vi "beta-3.1.0.vi"(5 "Load":bool, 6 "Configure":bool, 7 "Output Configuration":T2={"Channel0"={"function"=enum."OFF", "scan end"=3.5, "scan begin"=0.0, "scan step"=0.0, "main input"=enum."DIO0", "sub input"=enum."DIO0", "boolean low"=3.5, "boolean high"=0.0}, "Channel1"={"function"=enum."OFF", "scan end"=3.5, "scan begin"=0.0, "scan step"=0.0, "main input"=enum."DIO0", "sub input"=enum."DIO0", "boolean low"=3.5, "boolean high"=0.0}, "Channel2"={"function"=enum."OFF", "scan end"=3.5, "scan begin"=0.0, "scan step"=0.0, "main input"=enum."DIO0", "sub input"=enum."DIO0", "boolean low"=3.5, "boolean high"=0.0}, "Channel3"={"function"=enum."OFF", "scan end"=3.5, "scan begin"=0.0, "scan step"=0.0, "main input"=enum."DIO0", "sub input"=enum."DIO0", "boolean low"=3.5, "boolean high"=0.0}, "Channel4"={"function"=enum."OFF", "scan end"=3.5, "scan begin"=0.0, "scan step"=0.0, "main input"=enum."DIO0", "sub input"=enum."DIO0", "boolean low"=3.5, "boolean high"=0.0}, "Channel5"={"function"=enum."OFF", "scan end"=3.5, "scan begin"=0.0, "scan step"=0.0, "main input"=enum."DIO0", "sub input"=enum."DIO0", "boolean low"=3.5, "boolean high"=0.0}, "Channel6"={"function"=enum."OFF", "scan end"=3.5, "scan begin"=0.0, "scan step"=0.0, "main input"=enum."DIO0", "sub input"=enum."DIO0", "boolean low"=3.5, "boolean high"=0.0}, "Channel7"={"function"=enum."OFF", "scan end"=3.5, "scan begin"=0.0, "scan step"=0.0, "main input"=enum."DIO0", "sub input"=enum."DIO0", "boolean low"=3.5, "boolean high"=0.0}, "Channel8"={"function"=enum."OFF", "scan end"=3.5, "scan begin"=0.0, "scan step"=0.0, "main input"=enum."DIO0", "sub input"=enum."DIO0", "boolean low"=3.5, "boolean high"=0.0}, "Channel9"={"function"=enum."OFF", "scan end"=3.5, "scan begin"=0.0, "scan step"=0.0, "main input"=enum."DIO0", "sub input"=enum."DIO0", "boolean low"=3.5, "boolean high"=0.0}, "Channel10"={"function"=enum."OFF", "scan end"=3.5, "scan begin"=0.0, "scan step"=0.0, "main input"=enum."DIO0", "sub input"=enum."DIO0", "boolean low"=3.5, "boolean high"=0.0}, "Channel11"={"function"=enum."OFF", "scan end"=3.5, "scan begin"=0.0, "scan step"=0.0, "main input"=enum."DIO0", "sub input"=enum."DIO0", "boolean low"=3.5, "boolean high"=0.0}, "Channel12"={"function"=enum."OFF", "scan end"=3.5, "scan begin"=0.0, "scan step"=0.0, "main input"=enum."DIO0", "sub input"=enum."DIO0", "boolean low"=3.5, "boolean high"=0.0}, "Channel13"={"function"=enum."OFF", "scan end"=3.5, "scan begin"=0.0, "scan step"=0.0, "main input"=enum."DIO0", "sub input"=enum."DIO0", "boolean low"=3.5, "boolean high"=0.0}, "Channel14"={"function"=enum."OFF", "scan end"=3.5, "scan begin"=0.0, "scan step"=0.0, "main input"=enum."DIO0", "sub input"=enum."DIO0", "boolean low"=3.5, "boolean high"=0.0}, "Channel15"={"function"=enum."OFF", "scan end"=3.5, "scan begin"=0.0, "scan step"=0.0, "main input"=enum."DIO0", "sub input"=enum."DIO0", "boolean low"=3.5, "boolean high"=0.0}} {"Channel15"."boolean high" format="%#_17g"; "Channel15"."boolean low" format="%#_17g"; "Channel15"."scan step" format="%#_17g"; "Channel15"."scan begin" format="%#_17g"; "Channel15"."scan end" format="%#_17g"; "Channel14"."boolean high" format="%#_17g"; "Channel14"."boolean low" format="%#_17g"; "Channel14"."scan step" format="%#_17g"; "Channel14"."scan begin" format="%#_17g"; "Channel14"."scan end" format="%#_17g"; "Channel13"."boolean high" format="%#_17g"; "Channel13"."boolean low" format="%#_17g"; "Channel13"."scan step" format="%#_17g"; "Channel13"."scan begin" format="%#_17g"; "Channel13"."scan end" format="%#_17g"; "Channel12"."boolean high" format="%#_17g"; "Channel12"."boolean low" format="%#_17g"; "Channel12"."scan step" format="%#_17g"; "Channel12"."scan begin" format="%#_17g"; "Channel12"."scan end" format="%#_17g"; "Channel11"."boolean high" format="%#_17g"; "Channel11"."boolean low" format="%#_17g"; "Channel11"."scan step" format="%#_17g"; "Channel11"."scan begin" format="%#_17g"; "Channel11"."scan end" format="%#_17g"; "Channel10"."boolean high" format="%#_17g"; "Channel10"."boolean low" format="%#_17g"; "Channel10"."scan step" format="%#_17g"; "Channel10"."scan begin" format="%#_17g"; "Channel10"."scan end" format="%#_17g"; "Channel9"."boolean high" format="%#_17g"; "Channel9"."boolean low" format="%#_17g"; "Channel9"."scan step" format="%#_17g"; "Channel9"."scan begin" format="%#_17g"; "Channel9"."scan end" format="%#_17g"; "Channel8"."boolean high" format="%#_17g"; "Channel8"."boolean low" format="%#_17g"; "Channel8"."scan step" format="%#_17g"; "Channel8"."scan begin" format="%#_17g"; "Channel8"."scan end" format="%#_17g"; "Channel7"."boolean high" format="%#_17g"; "Channel7"."boolean low" format="%#_17g"; "Channel7"."scan step" format="%#_17g"; "Channel7"."scan begin" format="%#_17g"; "Channel7"."scan end" format="%#_17g"; "Channel6"."boolean high" format="%#_17g"; "Channel6"."boolean low" format="%#_17g"; "Channel6"."scan step" format="%#_17g"; "Channel6"."scan begin" format="%#_17g"; "Channel6"."scan end" format="%#_17g"; "Channel5"."boolean high" format="%#_17g"; "Channel5"."boolean low" format="%#_17g"; "Channel5"."scan step" format="%#_17g"; "Channel5"."scan begin" format="%#_17g"; "Channel5"."scan end" format="%#_17g"; "Channel4"."boolean high" format="%#_17g"; "Channel4"."boolean low" format="%#_17g"; "Channel4"."scan step" format="%#_17g"; "Channel4"."scan begin" format="%#_17g"; "Channel4"."scan end" format="%#_17g"; "Channel3"."boolean high" format="%#_17g"; "Channel3"."boolean low" format="%#_17g"; "Channel3"."scan step" format="%#_17g"; "Channel3"."scan begin" format="%#_17g"; "Channel3"."scan end" format="%#_17g"; "Channel2"."boolean high" format="%#_17g"; "Channel2"."boolean low" format="%#_17g"; "Channel2"."scan step" format="%#_17g"; "Channel2"."scan begin" format="%#_17g"; "Channel2"."scan end" format="%#_17g"; "Channel1"."boolean high" format="%#_17g"; "Channel1"."boolean low" format="%#_17g"; "Channel1"."scan step" format="%#_17g"; "Channel1"."scan begin" format="%#_17g"; "Channel1"."scan end" format="%#_17g"; "Channel0"."boolean high" format="%#_17g"; "Channel0"."boolean low" format="%#_17g"; "Channel0"."scan step" format="%#_17g"; "Channel0"."scan begin" format="%#_17g"; "Channel0"."scan end" format="%#_17g"}) -> (0 "State":enum16{"Loading", "Running"}(ring), 4 "change indicator":T1)   [LabVIEW 2016]
uses:
  <vilib>/FPGAPlugInAG/cRIO-9063/niLvFpga_Open_cRIO-9063.vi
  <vilib>/rvi/interface/common/dynamic/niFpgaDynamicAddResources.vi
  <vilib>/Utility/error.llb/Error Cluster From Error Code.vi
  <vilib>/rvi/errors/niLvFpgaAdjustHostInterfaceError.vi
  <vilib>/FPGAPlugInAG/Dynamic/niLvFpga_Close_Dynamic.vi
  <vilib>/rvi/interface/nirviOpenFPGA/nirviOpenFPGA.xnode
  FPGA Bitfiles/multi-functionpr_FPGATarget_multi-function-f_bsn-gyeHrfY.lvbitx
  <vilib>/rvi/interface/nirviReadWriteControl/nirviReadWriteControl.xnode
  <vilib>/rvi/interface/nirviCloseFPGA/nirviCloseFPGA.xnode
  NiFpgaLv.dll
  <vilib>/rvi/interface/Simulation/niFpgaSimulationCallBeginRW.vi
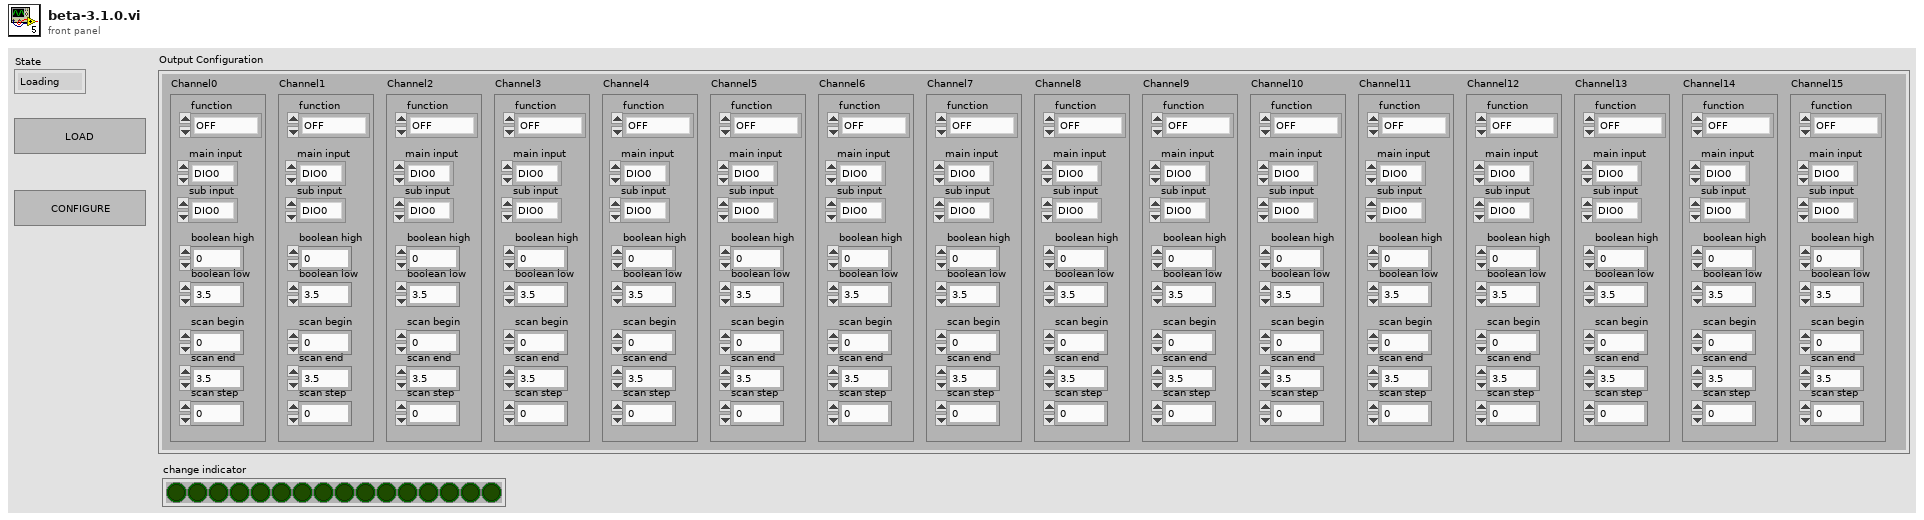
[diagram p1: front panel]
types:
  T1 = cluster{bool, bool, bool, bool, bool, bool, bool, bool, bool, bool, bool, bool, bool, bool, bool, bool}
  T2 = cluster{"Channel0":cluster{"function":enum16{"OFF", "SWITCH", "AND GATE", "OR GATE", "ITERATION"}, "scan end":sgl, "scan begin":sgl, "scan step":sgl, "main input":enum16{"DIO0", "DIO1", "DIO2", "DIO3", "DIO4", "DIO5", "DIO6", "DIO7", "DIO8", "DIO9", "DIO10", "DIO11", "DIO12", "DIO13", "DIO14", "DIO15", "DIO16", "DIO17", "DIO18", "DIO19", "DIO20", "DIO21", "DIO22", "DIO23", "DIO24", "DIO25", "DIO26", "DIO27", "DIO28", "DIO29", "DIO30", "DIO31"}, "sub input":enum16{"DIO0", "DIO1", "DIO2", "DIO3", "DIO4", "DIO5", "DIO6", "DIO7", "DIO8", "DIO9", "DIO10", "DIO11", "DIO12", "DIO13", "DIO14", "DIO15", "DIO16", "DIO17", "DIO18", "DIO19", "DIO20", "DIO21", "DIO22", "DIO23", "DIO24", "DIO25", "DIO26", "DIO27", "DIO28", "DIO29", "DIO30", "DIO31"}, "boolean low":sgl, "boolean high":sgl}, "Channel1":cluster{"function":enum16{"OFF", "SWITCH", "AND GATE", "OR GATE", "ITERATION"}, "scan end":sgl, "scan begin":sgl, "scan step":sgl, "main input":enum16{"DIO0", "DIO1", "DIO2", "DIO3", "DIO4", "DIO5", "DIO6", "DIO7", "DIO8", "DIO9", "DIO10", "DIO11", "DIO12", "DIO13", "DIO14", "DIO15", "DIO16", "DIO17", "DIO18", "DIO19", "DIO20", "DIO21", "DIO22", "DIO23", "DIO24", "DIO25", "DIO26", "DIO27", "DIO28", "DIO29", "DIO30", "DIO31"}, "sub input":enum16{"DIO0", "DIO1", "DIO2", "DIO3", "DIO4", "DIO5", "DIO6", "DIO7", "DIO8", "DIO9", "DIO10", "DIO11", "DIO12", "DIO13", "DIO14", "DIO15", "DIO16", "DIO17", "DIO18", "DIO19", "DIO20", "DIO21", "DIO22", "DIO23", "DIO24", "DIO25", "DIO26", "DIO27", "DIO28", "DIO29", "DIO30", "DIO31"}, "boolean low":sgl, "boolean high":sgl}, "Channel2":cluster{"function":enum16{"OFF", "SWITCH", "AND GATE", "OR GATE", "ITERATION"}, "scan end":sgl, "scan begin":sgl, "scan step":sgl, "main input":enum16{"DIO0", "DIO1", "DIO2", "DIO3", "DIO4", "DIO5", "DIO6", "DIO7", "DIO8", "DIO9", "DIO10", "DIO11", "DIO12", "DIO13", "DIO14", "DIO15", "DIO16", "DIO17", "DIO18", "DIO19", "DIO20", "DIO21", "DIO22", "DIO23", "DIO24", "DIO25", "DIO26", "DIO27", "DIO28", "DIO29", "DIO30", "DIO31"}, "sub input":enum16{"DIO0", "DIO1", "DIO2", "DIO3", "DIO4", "DIO5", "DIO6", "DIO7", "DIO8", "DIO9", "DIO10", "DIO11", "DIO12", "DIO13", "DIO14", "DIO15", "DIO16", "DIO17", "DIO18", "DIO19", "DIO20", "DIO21", "DIO22", "DIO23", "DIO24", "DIO25", "DIO26", "DIO27", "DIO28", "DIO29", "DIO30", "DIO31"}, "boolean low":sgl, "boolean high":sgl}, "Channel3":cluster{"function":enum16{"OFF", "SWITCH", "AND GATE", "OR GATE", "ITERATION"}, "scan end":sgl, "scan begin":sgl, "scan step":sgl, "main input":enum16{"DIO0", "DIO1", "DIO2", "DIO3", "DIO4", "DIO5", "DIO6", "DIO7", "DIO8", "DIO9", "DIO10", "DIO11", "DIO12", "DIO13", "DIO14", "DIO15", "DIO16", "DIO17", "DIO18", "DIO19", "DIO20", "DIO21", "DIO22", "DIO23", "DIO24", "DIO25", "DIO26", "DIO27", "DIO28", "DIO29", "DIO30", "DIO31"}, "sub input":enum16{"DIO0", "DIO1", "DIO2", "DIO3", "DIO4", "DIO5", "DIO6", "DIO7", "DIO8", "DIO9", "DIO10", "DIO11", "DIO12", "DIO13", "DIO14", "DIO15", "DIO16", "DIO17", "DIO18", "DIO19", "DIO20", "DIO21", "DIO22", "DIO23", "DIO24", "DIO25", "DIO26", "DIO27", "DIO28", "DIO29", "DIO30", "DIO31"}, "boolean low":sgl, "boolean high":sgl}, "Channel4":cluster{"function":enum16{"OFF", "SWITCH", "AND GATE", "OR GATE", "ITERATION"}, "scan end":sgl, "scan begin":sgl, "scan step":sgl, "main input":enum16{"DIO0", "DIO1", "DIO2", "DIO3", "DIO4", "DIO5", "DIO6", "DIO7", "DIO8", "DIO9", "DIO10", "DIO11", "DIO12", "DIO13", "DIO14", "DIO15", "DIO16", "DIO17", "DIO18", "DIO19", "DIO20", "DIO21", "DIO22", "DIO23", "DIO24", "DIO25", "DIO26", "DIO27", "DIO28", "DIO29", "DIO30", "DIO31"}, "sub input":enum16{"DIO0", "DIO1", "DIO2", "DIO3", "DIO4", "DIO5", "DIO6", "DIO7", "DIO8", "DIO9", "DIO10", "DIO11", "DIO12", "DIO13", "DIO14", "DIO15", "DIO16", "DIO17", "DIO18", "DIO19", "DIO20", "DIO21", "DIO22", "DIO23", "DIO24", "DIO25", "DIO26", "DIO27", "DIO28", "DIO29", "DIO30", "DIO31"}, "boolean low":sgl, "boolean high":sgl}, "Channel5":cluster{"function":enum16{"OFF", "SWITCH", "AND GATE", "OR GATE", "ITERATION"}, "scan end":sgl, "scan begin":sgl, "scan step":sgl, "main input":enum16{"DIO0", "DIO1", "DIO2", "DIO3", "DIO4", "DIO5", "DIO6", "DIO7", "DIO8", "DIO9", "DIO10", "DIO11", "DIO12", "DIO13", "DIO14", "DIO15", "DIO16", "DIO17", "DIO18", "DIO19", "DIO20", "DIO21", "DIO22", "DIO23", "DIO24", "DIO25", "DIO26", "DIO27", "DIO28", "DIO29", "DIO30", "DIO31"}, "sub input":enum16{"DIO0", "DIO1", "DIO2", "DIO3", "DIO4", "DIO5", "DIO6", "DIO7", "DIO8", "DIO9", "DIO10", "DIO11", "DIO12", "DIO13", "DIO14", "DIO15", "DIO16", "DIO17", "DIO18", "DIO19", "DIO20", "DIO21", "DIO22", "DIO23", "DIO24", "DIO25", "DIO26", "DIO27", "DIO28", "DIO29", "DIO30", "DIO31"}, "boolean low":sgl, "boolean high":sgl}, "Channel6":cluster{"function":enum16{"OFF", "SWITCH", "AND GATE", "OR GATE", "ITERATION"}, "scan end":sgl, "scan begin":sgl, "scan step":sgl, "main input":enum16{"DIO0", "DIO1", "DIO2", "DIO3", "DIO4", "DIO5", "DIO6", "DIO7", "DIO8", "DIO9", "DIO10", "DIO11", "DIO12", "DIO13", "DIO14", "DIO15", "DIO16", "DIO17", "DIO18", "DIO19", "DIO20", "DIO21", "DIO22", "DIO23", "DIO24", "DIO25", "DIO26", "DIO27", "DIO28", "DIO29", "DIO30", "DIO31"}, "sub input":enum16{"DIO0", "DIO1", "DIO2", "DIO3", "DIO4", "DIO5", "DIO6", "DIO7", "DIO8", "DIO9", "DIO10", "DIO11", "DIO12", "DIO13", "DIO14", "DIO15", "DIO16", "DIO17", "DIO18", "DIO19", "DIO20", "DIO21", "DIO22", "DIO23", "DIO24", "DIO25", "DIO26", "DIO27", "DIO28", "DIO29", "DIO30", "DIO31"}, "boolean low":sgl, "boolean high":sgl}, "Channel7":cluster{"function":enum16{"OFF", "SWITCH", "AND GATE", "OR GATE", "ITERATION"}, "scan end":sgl, "scan begin":sgl, "scan step":sgl, "main input":enum16{"DIO0", "DIO1", "DIO2", "DIO3", "DIO4", "DIO5", "DIO6", "DIO7", "DIO8", "DIO9", "DIO10", "DIO11", "DIO12", "DIO13", "DIO14", "DIO15", "DIO16", "DIO17", "DIO18", "DIO19", "DIO20", "DIO21", "DIO22", "DIO23", "DIO24", "DIO25", "DIO26", "DIO27", "DIO28", "DIO29", "DIO30", "DIO31"}, "sub input":enum16{"DIO0", "DIO1", "DIO2", "DIO3", "DIO4", "DIO5", "DIO6", "DIO7", "DIO8", "DIO9", "DIO10", "DIO11", "DIO12", "DIO13", "DIO14", "DIO15", "DIO16", "DIO17", "DIO18", "DIO19", "DIO20", "DIO21", "DIO22", "DIO23", "DIO24", "DIO25", "DIO26", "DIO27", "DIO28", "DIO29", "DIO30", "DIO31"}, "boolean low":sgl, "boolean high":sgl}, "Channel8":cluster{"function":enum16{"OFF", "SWITCH", "AND GATE", "OR GATE", "ITERATION"}, "scan end":sgl, "scan begin":sgl, "scan step":sgl, "main input":enum16{"DIO0", "DIO1", "DIO2", "DIO3", "DIO4", "DIO5", "DIO6", "DIO7", "DIO8", "DIO9", "DIO10", "DIO11", "DIO12", "DIO13", "DIO14", "DIO15", "DIO16", "DIO17", "DIO18", "DIO19", "DIO20", "DIO21", "DIO22", "DIO23", "DIO24", "DIO25", "DIO26", "DIO27", "DIO28", "DIO29", "DIO30", "DIO31"}, "sub input":enum16{"DIO0", "DIO1", "DIO2", "DIO3", "DIO4", "DIO5", "DIO6", "DIO7", "DIO8", "DIO9", "DIO10", "DIO11", "DIO12", "DIO13", "DIO14", "DIO15", "DIO16", "DIO17", "DIO18", "DIO19", "DIO20", "DIO21", "DIO22", "DIO23", "DIO24", "DIO25", "DIO26", "DIO27", "DIO28", "DIO29", "DIO30", "DIO31"}, "boolean low":sgl, "boolean high":sgl}, "Channel9":cluster{"function":enum16{"OFF", "SWITCH", "AND GATE", "OR GATE", "ITERATION"}, "scan end":sgl, "scan begin":sgl, "scan step":sgl, "main input":enum16{"DIO0", "DIO1", "DIO2", "DIO3", "DIO4", "DIO5", "DIO6", "DIO7", "DIO8", "DIO9", "DIO10", "DIO11", "DIO12", "DIO13", "DIO14", "DIO15", "DIO16", "DIO17", "DIO18", "DIO19", "DIO20", "DIO21", "DIO22", "DIO23", "DIO24", "DIO25", "DIO26", "DIO27", "DIO28", "DIO29", "DIO30", "DIO31"}, "sub input":enum16{"DIO0", "DIO1", "DIO2", "DIO3", "DIO4", "DIO5", "DIO6", "DIO7", "DIO8", "DIO9", "DIO10", "DIO11", "DIO12", "DIO13", "DIO14", "DIO15", "DIO16", "DIO17", "DIO18", "DIO19", "DIO20", "DIO21", "DIO22", "DIO23", "DIO24", "DIO25", "DIO26", "DIO27", "DIO28", "DIO29", "DIO30", "DIO31"}, "boolean low":sgl, "boolean high":sgl}, "Channel10":cluster{"function":enum16{"OFF", "SWITCH", "AND GATE", "OR GATE", "ITERATION"}, "scan end":sgl, "scan begin":sgl, "scan step":sgl, "main input":enum16{"DIO0", "DIO1", "DIO2", "DIO3", "DIO4", "DIO5", "DIO6", "DIO7", "DIO8", "DIO9", "DIO10", "DIO11", "DIO12", "DIO13", "DIO14", "DIO15", "DIO16", "DIO17", "DIO18", "DIO19", "DIO20", "DIO21", "DIO22", "DIO23", "DIO24", "DIO25", "DIO26", "DIO27", "DIO28", "DIO29", "DIO30", "DIO31"}, "sub input":enum16{"DIO0", "DIO1", "DIO2", "DIO3", "DIO4", "DIO5", "DIO6", "DIO7", "DIO8", "DIO9", "DIO10", "DIO11", "DIO12", "DIO13", "DIO14", "DIO15", "DIO16", "DIO17", "DIO18", "DIO19", "DIO20", "DIO21", "DIO22", "DIO23", "DIO24", "DIO25", "DIO26", "DIO27", "DIO28", "DIO29", "DIO30", "DIO31"}, "boolean low":sgl, "boolean high":sgl}, "Channel11":cluster{"function":enum16{"OFF", "SWITCH", "AND GATE", "OR GATE", "ITERATION"}, "scan end":sgl, "scan begin":sgl, "scan step":sgl, "main input":enum16{"DIO0", "DIO1", "DIO2", "DIO3", "DIO4", "DIO5", "DIO6", "DIO7", "DIO8", "DIO9", "DIO10", "DIO11", "DIO12", "DIO13", "DIO14", "DIO15", "DIO16", "DIO17", "DIO18", "DIO19", "DIO20", "DIO21", "DIO22", "DIO23", "DIO24", "DIO25", "DIO26", "DIO27", "DIO28", "DIO29", "DIO30", "DIO31"}, "sub input":enum16{"DIO0", "DIO1", "DIO2", "DIO3", "DIO4", "DIO5", "DIO6", "DIO7", "DIO8", "DIO9", "DIO10", "DIO11", "DIO12", "DIO13", "DIO14", "DIO15", "DIO16", "DIO17", "DIO18", "DIO19", "DIO20", "DIO21", "DIO22", "DIO23", "DIO24", "DIO25", "DIO26", "DIO27", "DIO28", "DIO29", "DIO30", "DIO31"}, "boolean low":sgl, "boolean high":sgl}, "Channel12":cluster{"function":enum16{"OFF", "SWITCH", "AND GATE", "OR GATE", "ITERATION"}, "scan end":sgl, "scan begin":sgl, "scan step":sgl, "main input":enum16{"DIO0", "DIO1", "DIO2", "DIO3", "DIO4", "DIO5", "DIO6", "DIO7", "DIO8", "DIO9", "DIO10", "DIO11", "DIO12", "DIO13", "DIO14", "DIO15", "DIO16", "DIO17", "DIO18", "DIO19", "DIO20", "DIO21", "DIO22", "DIO23", "DIO24", "DIO25", "DIO26", "DIO27", "DIO28", "DIO29", "DIO30", "DIO31"}, "sub input":enum16{"DIO0", "DIO1", "DIO2", "DIO3", "DIO4", "DIO5", "DIO6", "DIO7", "DIO8", "DIO9", "DIO10", "DIO11", "DIO12", "DIO13", "DIO14", "DIO15", "DIO16", "DIO17", "DIO18", "DIO19", "DIO20", "DIO21", "DIO22", "DIO23", "DIO24", "DIO25", "DIO26", "DIO27", "DIO28", "DIO29", "DIO30", "DIO31"}, "boolean low":sgl, "boolean high":sgl}, "Channel13":cluster{"function":enum16{"OFF", "SWITCH", "AND GATE", "OR GATE", "ITERATION"}, "scan end":sgl, "scan begin":sgl, "scan step":sgl, "main input":enum16{"DIO0", "DIO1", "DIO2", "DIO3", "DIO4", "DIO5", "DIO6", "DIO7", "DIO8", "DIO9", "DIO10", "DIO11", "DIO12", "DIO13", "DIO14", "DIO15", "DIO16", "DIO17", "DIO18", "DIO19", "DIO20", "DIO21", "DIO22", "DIO23", "DIO24", "DIO25", "DIO26", "DIO27", "DIO28", "DIO29", "DIO30", "DIO31"}, "sub input":enum16{"DIO0", "DIO1", "DIO2", "DIO3", "DIO4", "DIO5", "DIO6", "DIO7", "DIO8", "DIO9", "DIO10", "DIO11", "DIO12", "DIO13", "DIO14", "DIO15", "DIO16", "DIO17", "DIO18", "DIO19", "DIO20", "DIO21", "DIO22", "DIO23", "DIO24", "DIO25", "DIO26", "DIO27", "DIO28", "DIO29", "DIO30", "DIO31"}, "boolean low":sgl, "boolean high":sgl}, "Channel14":cluster{"function":enum16{"OFF", "SWITCH", "AND GATE", "OR GATE", "ITERATION"}, "scan end":sgl, "scan begin":sgl, "scan step":sgl, "main input":enum16{"DIO0", "DIO1", "DIO2", "DIO3", "DIO4", "DIO5", "DIO6", "DIO7", "DIO8", "DIO9", "DIO10", "DIO11", "DIO12", "DIO13", "DIO14", "DIO15", "DIO16", "DIO17", "DIO18", "DIO19", "DIO20", "DIO21", "DIO22", "DIO23", "DIO24", "DIO25", "DIO26", "DIO27", "DIO28", "DIO29", "DIO30", "DIO31"}, "sub input":enum16{"DIO0", "DIO1", "DIO2", "DIO3", "DIO4", "DIO5", "DIO6", "DIO7", "DIO8", "DIO9", "DIO10", "DIO11", "DIO12", "DIO13", "DIO14", "DIO15", "DIO16", "DIO17", "DIO18", "DIO19", "DIO20", "DIO21", "DIO22", "DIO23", "DIO24", "DIO25", "DIO26", "DIO27", "DIO28", "DIO29", "DIO30", "DIO31"}, "boolean low":sgl, "boolean high":sgl}, "Channel15":cluster{"function":enum16{"OFF", "SWITCH", "AND GATE", "OR GATE", "ITERATION"}, "scan end":sgl, "scan begin":sgl, "scan step":sgl, "main input":enum16{"DIO0", "DIO1", "DIO2", "DIO3", "DIO4", "DIO5", "DIO6", "DIO7", "DIO8", "DIO9", "DIO10", "DIO11", "DIO12", "DIO13", "DIO14", "DIO15", "DIO16", "DIO17", "DIO18", "DIO19", "DIO20", "DIO21", "DIO22", "DIO23", "DIO24", "DIO25", "DIO26", "DIO27", "DIO28", "DIO29", "DIO30", "DIO31"}, "sub input":enum16{"DIO0", "DIO1", "DIO2", "DIO3", "DIO4", "DIO5", "DIO6", "DIO7", "DIO8", "DIO9", "DIO10", "DIO11", "DIO12", "DIO13", "DIO14", "DIO15", "DIO16", "DIO17", "DIO18", "DIO19", "DIO20", "DIO21", "DIO22", "DIO23", "DIO24", "DIO25", "DIO26", "DIO27", "DIO28", "DIO29", "DIO30", "DIO31"}, "boolean low":sgl, "boolean high":sgl}}
  T3 = cluster{"Channel0":cluster{"function":bool, "scan end":bool, "scan begin":bool, "scan step":bool, "main input":bool, "sub input":bool, "boolean low":bool, "boolean high":bool}, "Channel1":cluster{"function":bool, "scan end":bool, "scan begin":bool, "scan step":bool, "main input":bool, "sub input":bool, "boolean low":bool, "boolean high":bool}, "Channel2":cluster{"function":bool, "scan end":bool, "scan begin":bool, "scan step":bool, "main input":bool, "sub input":bool, "boolean low":bool, "boolean high":bool}, "Channel3":cluster{"function":bool, "scan end":bool, "scan begin":bool, "scan step":bool, "main input":bool, "sub input":bool, "boolean low":bool, "boolean high":bool}, "Channel4":cluster{"function":bool, "scan end":bool, "scan begin":bool, "scan step":bool, "main input":bool, "sub input":bool, "boolean low":bool, "boolean high":bool}, "Channel5":cluster{"function":bool, "scan end":bool, "scan begin":bool, "scan step":bool, "main input":bool, "sub input":bool, "boolean low":bool, "boolean high":bool}, "Channel6":cluster{"function":bool, "scan end":bool, "scan begin":bool, "scan step":bool, "main input":bool, "sub input":bool, "boolean low":bool, "boolean high":bool}, "Channel7":cluster{"function":bool, "scan end":bool, "scan begin":bool, "scan step":bool, "main input":bool, "sub input":bool, "boolean low":bool, "boolean high":bool}, "Channel8":cluster{"function":bool, "scan end":bool, "scan begin":bool, "scan step":bool, "main input":bool, "sub input":bool, "boolean low":bool, "boolean high":bool}, "Channel9":cluster{"function":bool, "scan end":bool, "scan begin":bool, "scan step":bool, "main input":bool, "sub input":bool, "boolean low":bool, "boolean high":bool}, "Channel10":cluster{"function":bool, "scan end":bool, "scan begin":bool, "scan step":bool, "main input":bool, "sub input":bool, "boolean low":bool, "boolean high":bool}, "Channel11":cluster{"function":bool, "scan end":bool, "scan begin":bool, "scan step":bool, "main input":bool, "sub input":bool, "boolean low":bool, "boolean high":bool}, "Channel12":cluster{"function":bool, "scan end":bool, "scan begin":bool, "scan step":bool, "main input":bool, "sub input":bool, "boolean low":bool, "boolean high":bool}, "Channel13":cluster{"function":bool, "scan end":bool, "scan begin":bool, "scan step":bool, "main input":bool, "sub input":bool, "boolean low":bool, "boolean high":bool}, "Channel14":cluster{"function":bool, "scan end":bool, "scan begin":bool, "scan step":bool, "main input":bool, "sub input":bool, "boolean low":bool, "boolean high":bool}, "Channel15":cluster{"function":bool, "scan end":bool, "scan begin":bool, "scan step":bool, "main input":bool, "sub input":bool, "boolean low":bool, "boolean high":bool}}
  T4 = cluster{"function":bool, "scan end":bool, "scan begin":bool, "scan step":bool, "main input":bool, "sub input":bool, "boolean low":bool, "boolean high":bool}
  T5 = cluster{"function":enum16{"OFF", "SWITCH", "AND GATE", "OR GATE", "ITERATION"}, "scan end":sgl, "scan begin":sgl, "scan step":sgl, "main input":enum16{"DIO0", "DIO1", "DIO2", "DIO3", "DIO4", "DIO5", "DIO6", "DIO7", "DIO8", "DIO9", "DIO10", "DIO11", "DIO12", "DIO13", "DIO14", "DIO15", "DIO16", "DIO17", "DIO18", "DIO19", "DIO20", "DIO21", "DIO22", "DIO23", "DIO24", "DIO25", "DIO26", "DIO27", "DIO28", "DIO29", "DIO30", "DIO31"}, "sub input":enum16{"DIO0", "DIO1", "DIO2", "DIO3", "DIO4", "DIO5", "DIO6", "DIO7", "DIO8", "DIO9", "DIO10", "DIO11", "DIO12", "DIO13", "DIO14", "DIO15", "DIO16", "DIO17", "DIO18", "DIO19", "DIO20", "DIO21", "DIO22", "DIO23", "DIO24", "DIO25", "DIO26", "DIO27", "DIO28", "DIO29", "DIO30", "DIO31"}, "boolean low":sgl, "boolean high":sgl}
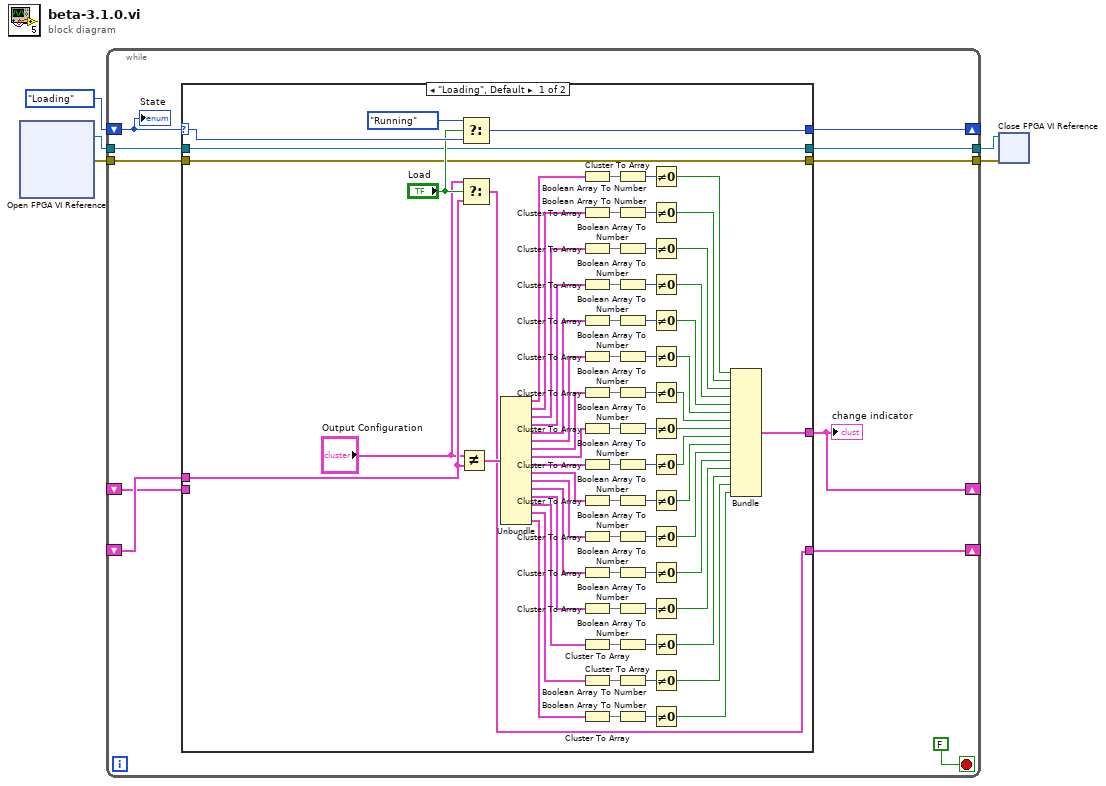
[diagram p0: block diagram]
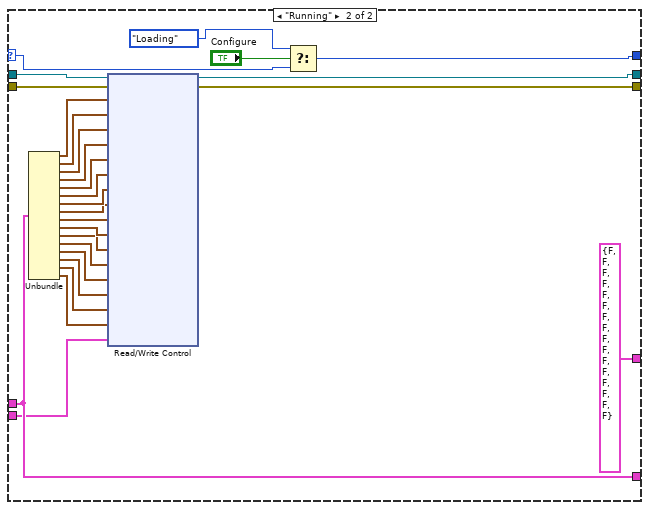
[diagram p2: hidden frame]
diagram:
  n1 = xnode "Open FPGA VI Reference"() -> ("FPGA VI Reference Out"=w4:refnum<k20>, "error out"=w3:errorcluster)  [unwired: 2 in]
  n2 = while {
    shift-right: [w13] -> _
    shift-left: _ -> [w12]
    shift-right: [w15] -> _
    shift-left: enum16{"Loading", "Running"}."Loading" ("State") -> [w14]
    shift-right: [w11] -> _
    shift-left: _ -> [w6]
    tunnel: w4 -> [w10]
    tunnel: w3 -> [w9]
    tunnel: [w8] -> w2
    tunnel: [w7] -> w1
    stop <- FALSE stop-if-true
    n3 = case shown="\"Loading\", Default" w14 {
      selector: w14 -> [w91 w115]
      tunnel: [w90 w117] -> w15
      tunnel: [w84 w109] -> w13
      tunnel: w12 -> [w86 w109]
      tunnel: [w19 T1 {FALSE, FALSE, FALSE, FALSE, FALSE, FALSE, FALSE, FALSE, FALSE, FALSE, FALSE, FALSE, FALSE, FALSE, FALSE, FALSE}] -> w11
      tunnel: w10 -> [w18 w113]
      tunnel: w9 -> [w17 w112]
      tunnel: [w18 w111] -> w8
      tunnel: [w17 w110] -> w7
      tunnel: w6 -> [_ w92]
      frame "Loading", Default {
        n4 = Not Equal?(x="Output Configuration", y=w86) -> (x != y?=w88:T3)
        n5 = Select(t=enum16{"Loading", "Running"}."Running", s="Load", f=w91) -> (s? t:f=w90:enum16{"Loading", "Running"})
        n6 = Select(t="Output Configuration", s="Load", f=w86) -> (s? t:f=w84:T2)
        n7 = Unbundle(w88) -> ("Channel0"=w51:T4, "Channel1"=w50:T4, "Channel2"=w49:T4, "Channel3"=w48:T4, "Channel4"=w47:T4, "Channel5"=w46:T4, "Channel6"=w45:T4, "Channel7"=w44:T4, "Channel8"=w43:T4, "Channel9"=w42:T4, "Channel10"=w41:T4, "Channel11"=w40:T4, "Channel12"=w39:T4, "Channel13"=w38:T4, "Channel14"=w37:T4, "Channel15"=w36:T4)
        n8 = Cluster To Array(cluster=w51) -> (array=w61:bool[])
        n9 = Cluster To Array(cluster=w50) -> (array=w63:bool[])
        n10 = Cluster To Array(cluster=w49) -> (array=w65:bool[])
        n11 = Cluster To Array(cluster=w48) -> (array=w67:bool[])
        n12 = Cluster To Array(cluster=w47) -> (array=w69:bool[])
        n13 = Cluster To Array(cluster=w46) -> (array=w83:bool[])
        n14 = Cluster To Array(cluster=w45) -> (array=w79:bool[])
        n15 = Cluster To Array(cluster=w44) -> (array=w81:bool[])
        n16 = Cluster To Array(cluster=w43) -> (array=w77:bool[])
        n17 = Cluster To Array(cluster=w42) -> (array=w75:bool[])
        n18 = Cluster To Array(cluster=w41) -> (array=w73:bool[])
        n19 = Cluster To Array(cluster=w40) -> (array=w71:bool[])
        n20 = Cluster To Array(cluster=w39) -> (array=w59:bool[])
        n21 = Cluster To Array(cluster=w38) -> (array=w57:bool[])
        n22 = Cluster To Array(cluster=w37) -> (array=w55:bool[])
        n23 = Cluster To Array(cluster=w36) -> (array=w53:bool[])
        n24 = Boolean Array To Number(Boolean array=w61) -> (number=w60:u32)
        n25 = Boolean Array To Number(Boolean array=w63) -> (number=w62:u32)
        n26 = Boolean Array To Number(Boolean array=w65) -> (number=w64:u32)
        n27 = Boolean Array To Number(Boolean array=w67) -> (number=w66:u32)
        n28 = Boolean Array To Number(Boolean array=w69) -> (number=w68:u32)
        n29 = Boolean Array To Number(Boolean array=w83) -> (number=w82:u32)
        n30 = Boolean Array To Number(Boolean array=w79) -> (number=w78:u32)
        n31 = Boolean Array To Number(Boolean array=w81) -> (number=w80:u32)
        n32 = Boolean Array To Number(Boolean array=w77) -> (number=w76:u32)
        n33 = Boolean Array To Number(Boolean array=w75) -> (number=w74:u32)
        n34 = Boolean Array To Number(Boolean array=w73) -> (number=w72:u32)
        n35 = Boolean Array To Number(Boolean array=w71) -> (number=w70:u32)
        n36 = Boolean Array To Number(Boolean array=w59) -> (number=w58:u32)
        n37 = Boolean Array To Number(Boolean array=w57) -> (number=w56:u32)
        n38 = Boolean Array To Number(Boolean array=w55) -> (number=w54:u32)
        n39 = Boolean Array To Number(Boolean array=w53) -> (number=w52:u32)
        n40 = Not Equal To 0?(x=w60) -> (x != 0?=w35:bool)
        n41 = Not Equal To 0?(x=w62) -> (x != 0?=w34:bool)
        n42 = Not Equal To 0?(x=w64) -> (x != 0?=w33:bool)
        n43 = Not Equal To 0?(x=w66) -> (x != 0?=w32:bool)
        n44 = Not Equal To 0?(x=w68) -> (x != 0?=w31:bool)
        n45 = Not Equal To 0?(x=w82) -> (x != 0?=w30:bool)
        n46 = Not Equal To 0?(x=w78) -> (x != 0?=w29:bool)
        n47 = Not Equal To 0?(x=w80) -> (x != 0?=w28:bool)
        n48 = Not Equal To 0?(x=w76) -> (x != 0?=w27:bool)
        n49 = Not Equal To 0?(x=w74) -> (x != 0?=w26:bool)
        n50 = Not Equal To 0?(x=w72) -> (x != 0?=w25:bool)
        n51 = Not Equal To 0?(x=w70) -> (x != 0?=w24:bool)
        n52 = Not Equal To 0?(x=w58) -> (x != 0?=w23:bool)
        n53 = Not Equal To 0?(x=w56) -> (x != 0?=w22:bool)
        n54 = Not Equal To 0?(x=w54) -> (x != 0?=w21:bool)
        n55 = Not Equal To 0?(x=w52) -> (x != 0?=w20:bool)
        n56 = Bundle(w35, w34, w33, w32, w31, w30, w29, w28, w27, w26, w25, w24, w23, w22, w21, w20) -> (w19:T1)  [unwired: 1 in]
      }
      frame "Running" {
        n57 = Unbundle(w109) -> ("Channel0"=w108:T5, "Channel1"=w107:T5, "Channel2"=w106:T5, "Channel3"=w105:T5, "Channel4"=w104:T5, "Channel5"=w103:T5, "Channel6"=w102:T5, "Channel7"=w101:T5, "Channel8"=w100:T5, "Channel9"=w99:T5, "Channel10"=w98:T5, "Channel11"=w97:T5, "Channel12"=w96:T5, "Channel13"=w95:T5, "Channel14"=w94:T5, "Channel15"=w93:T5)
        n58 = xnode "Read/Write Control"("FPGA VI Reference In"=w113, "error in"=w112, "Channel0"=w108, "Channel1"=w107, "Channel2"=w106, "Channel3"=w105, "Channel4"=w104, "Channel5"=w103, "Channel6"=w102, "Channel7"=w101, "Channel8"=w100, "Channel9"=w99, "Channel10"=w98, "Channel11"=w97, "Channel12"=w96, "Channel13"=w95, "Channel14"=w94, "Channel15"=w93, "Reset buttons"=w92) -> ("FPGA VI Reference Out"=w111:refnum<k20>, "error out"=w110:errorcluster)
        n59 = Select(t=enum16{"Loading", "Running"}."Loading", s="Configure", f=w115) -> (s? t:f=w117:enum16{"Loading", "Running"})
      }
    }
    "change indicator" <- w11
    "State" <- w14
  }
  n60 = xnode "Close FPGA VI Reference"("FPGA VI Reference In"=w2, "error in"=w1) -> ()  [unwired: 1 out]
